vi "Stop.vi"(8 "error in":errorcluster, 9 "timeout (-1)":i32=-1, 11 "Standard Engine in":refnum<class "synchronous engine runtime.lvclass">) -> (0 "error out":errorcluster, 3 "Standard Engine out":refnum<class "synchronous engine runtime.lvclass">)   [LabVIEW 2013, in "synchronous engine runtime.lvclass"]
uses:
  synchronous engine runtime.lvclass
  Commands.ctl
  synchronous engine runtime.lvclass/synchronous engine runtime.ctl
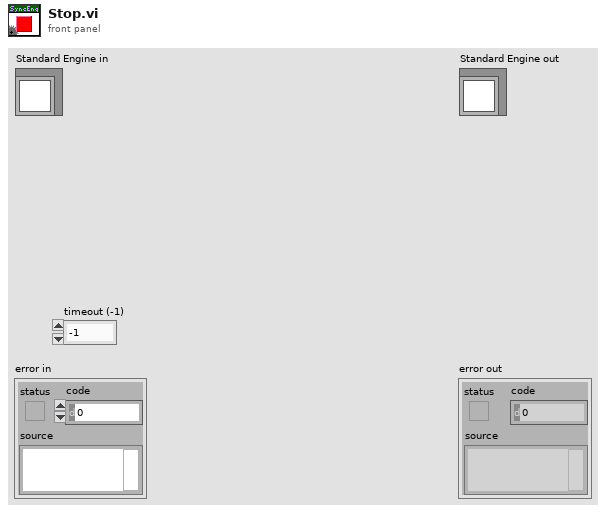
[diagram p1: front panel]
types:
  T1 = typedef "synchronous engine runtime.lvclass/Commands.ctl" = enum16{"Start", "Pause", "Safe State", "Normal", "Stop", "Shutdown"}
  T2 = typedef "synchronous engine runtime.lvclass/Engine VI Ref.ctl" = refnum<vi>
  T3 = typedef "synchronous engine runtime.lvclass/notifier.ctl" = cluster{"Engine State":T4, "error constant":errorcluster}
  T4 = typedef "Engine Runtime Interface.lvclass/Execution States.ctl" = enum16{"Init", "Pre-Operational", "Safe-Operational", "Operational", "Stopped"}
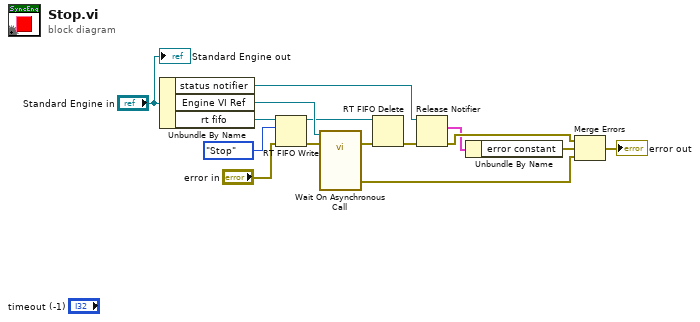
[diagram p0: block diagram]
diagram:
  n1 = Unbundle By Name("Standard Engine in") -> ("status notifier"=w6:refnum<notifier>, "Engine VI Ref"=w10:T2, "rt fifo"=w15:refnum<k33>)
  n2 = RT FIFO Write(0:w15, 1:Commands."Stop" ("element"), 3:"error in") -> (8:w8:refnum<k33>, 11:w13:errorcluster)  [unwired: 2 in, 2 out]
  n3 = call-by-ref "Wait On Asynchronous Call"(reference=w10, error in=w13) -> (error out=w11:errorcluster, 0:"error out"=w2:errorcluster)  [unwired: 11 in, 1 out]
  n4 = RT FIFO Delete(0:w8, 3:w11) -> (11:w9:errorcluster)  [unwired: 1 in]
  n5 = Release Notifier(notifier=w6, error in (no error)=w9) -> (last notification=w5:T3, error out=w7:errorcluster)  [unwired: 1 in, 1 out]
  n6 = Unbundle By Name(w5) -> ("error constant"=w3:errorcluster)
  n7 = Merge Errors(w7, w3, w2) -> (→"error out":errorcluster)
  "Standard Engine out" <- "Standard Engine in"
